vi "MALT Output Get Several.vi"(8 "error in":errorcluster, 9 "Block":i32, 10 "Address":i32, 11 "MALT FamilyCode":T1=enum."MALT132") -> (0 "error out":errorcluster, 3 "Status Map":u8[](array[numeric]) format="%02x")   [LabVIEW 2018, in "AltonTech MALT200817.lvlib"]
uses:
  <instrlib>/AltonTech MALT/AltonTech MALT200817.lvlib
  <instrlib>/AltonTech MALT/Public/Types/MALT Family Codes.ctl
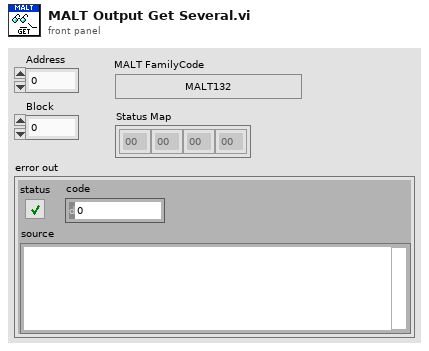
[diagram p1: front panel]
types:
  T1 = typedef "AltonTech MALT200817.lvlib/MALT Family Codes.ctl" = enum32{"-", "MALT40IO", "YAV904X8", "MALT132", "YAV91616", "MALT16PIN", "YAV90096", "YAV90HVT", "YAV90CLR", "YAV90128", "YAV90PNE", "YAVCANCON", "YAV91775", "YAV90XXX", "YAV90MMU", "H730050", "H710060", "H710061", "YAV90304", "MMI", "YAV90060", "MALT160T", "YAV90059", "Not Defined"}
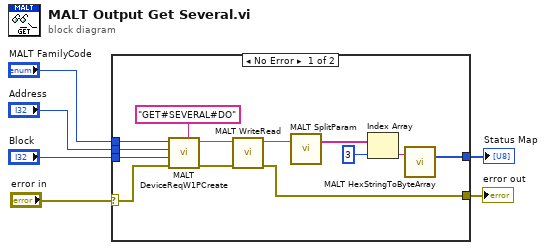
[diagram p0: block diagram]
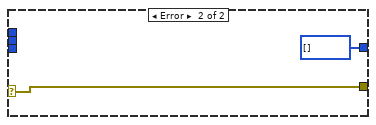
[diagram p2: hidden frame]
diagram:
  n1 = case shown="No Error" "error in" {
    selector: "error in" -> [w8 w20]
    tunnel: [w18 w20] -> w6
    tunnel: "Block" -> [w15 _]
    tunnel: "Address" -> [w14 _]
    tunnel: "MALT FamilyCode" -> [w11 _]
    tunnel: [w9 u8[] [] ("Bytes out")] -> w2
    frame No Error {
      n2 = call <instrlib>:"MALT DeviceReqW1PCreate.vi"("Cmd"="GET#SEVERAL#DO" ("cmd"), "error in"=w8, "Param1"=w15, "Address"=w14, "FamilyCode"=w11) -> ("error out"=w13:errorcluster, "Request"=w7:string)  [unwired: 4 in]
      n3 = call <instrlib>:"MALT WriteRead.vi"("error in"=w13, "Request"=w7) -> ("error out"=w18:errorcluster, "Response"=w19:string)  [unwired: 8 in]
      n4 = call <instrlib>:"MALT SplitParam.vi"("Line"=w19) -> ("Items"=w17:string[])  [unwired: 2 in]
      n5 = Index Array(array=w17, index=3) -> (element=w10:string)
      n6 = call <instrlib>:"MALT HexStringToByteArray.vi"("String in"=w10) -> ("Bytes out"=w9:u8[])  [unwired: 2 in]
    }
    frame Error {
    }
  }
  "error out" <- w6
  "Status Map" <- w2
